vi "General Polynomial Fit (Bisquare).vi"(0 "Y":dbl[](array[numeric]), 1 "polynomial order":i32=2, 2 "Coefficient Constraint":cluster{"order":i32, "coefficient":dbl}[](array[cluster]), 5 "X":dbl[](array[numeric]), 7 "Weight":dbl[](array[numeric]), 9 "tolerance":dbl=0.0001, 13 "algorithm":T1 items=["SVD", "Givens", "Givens2", "Householder", "LU Decomposition", "Cholesky", "SVD for Rank Deficient H"]) -> (4 "Best Polynomial Fit":dbl[](array[numeric]), 6 "Polynomial Coefficients":dbl[](array[numeric]), 14 "residue":dbl, 15 "error":i32)   [LabVIEW 2020, in "NI_AALPro.lvlib"]
uses:
  <vilib>/Analysis/NI_AALPro.lvlib
  <vilib>/Analysis/6fits.llb/General Linear Fit Algorithm.ctl
  <resource>/lvanlys.dll
panel:
  # "Bisquare General Polynomial Fit"
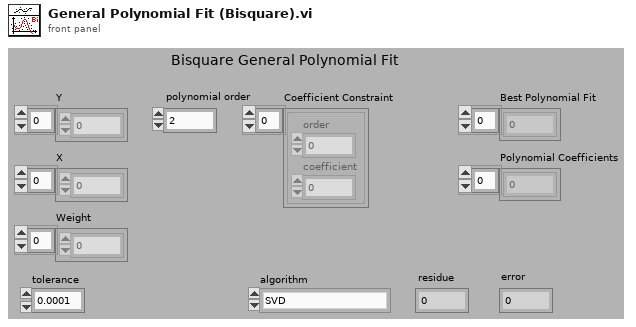
[diagram p1: front panel]
types:
  T1 = typedef "NI_AALPro.lvlib/General Linear Fit Algorithm.ctl" = u16
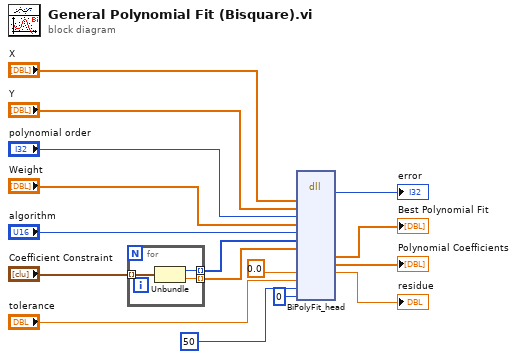
[diagram p0: block diagram]
diagram:
  n1 = for {
    tunnel: "Coefficient Constraint" -> [w19] mode=indexing
    tunnel: [w18] -> w16 mode=indexing
    tunnel: [w17] -> w15 mode=indexing
    n2 = Unbundle(w19) -> ("order"=w18:i32, "coefficient"=w17:dbl)
  }
  n3 = dll-call lib="e:/builds/penguin/labview/branches/2020/dev/dist/resource/lvanlys.*" fn="BiPolyFit_head"("xH"="X", "yH"="Y", "Order"="polynomial order", "weightH"="Weight", "algorithm"="algorithm", "specOrderH"=w16, "specCoefH"=w15, "mse"=0.0, "tolerance"="tolerance", "maxIter"=50, "iscoef"=0) -> ("return type"=→"error":i32, "BestFitH"=→"Best Polynomial Fit":dbl[], "CoefH"=→"Polynomial Coefficients":dbl[], "mse"=→"residue":dbl)  [unwired: 12 in, 5 out]
